vi "USBClose.vi"(8 "error in (no error)":errorcluster, 11 "USB":refnum<visa-resource-name>="USB0::0x1043::0x0000::NI-VISA-0::RAW") -> (0 "error out":errorcluster)   [LabVIEW 2011]
doc: "The vi are closing the specified USB connection."
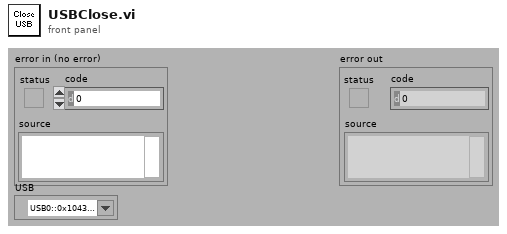
[diagram p1: front panel]
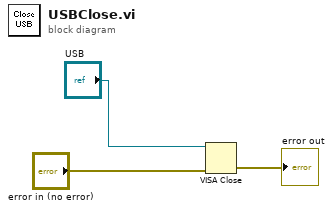
[diagram p0: block diagram]
diagram:
  n1 = VISA Close(VISA resource name="USB", error in (no error)="error in (no error)") -> (error out=→"error out":errorcluster)
